vi "Save File Get File Size.vi"(8 "Error In":errorcluster, 10 "File Size":dbl=5.0 format="%#_13g", 11 "Old path":path) -> (0 "Error Out":errorcluster, 2 "File Size MB":dbl, 3 "File Size Greater Than Limit":bool)   [LabVIEW 2016, in "Save File.lvlib"]
uses:
  Save File.lvlib
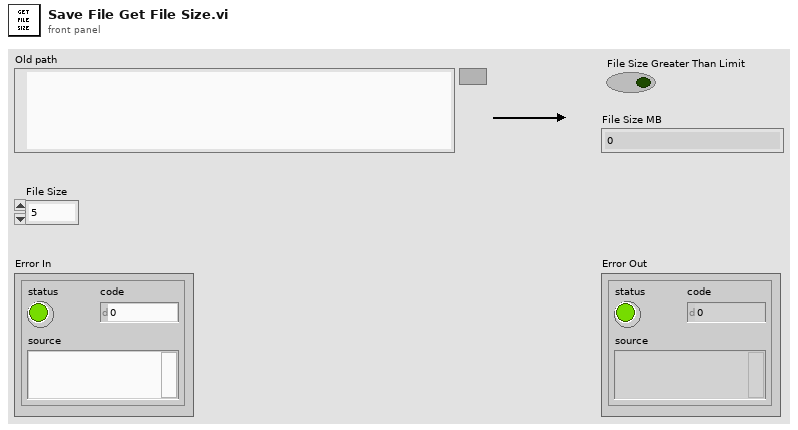
[diagram p1: front panel]
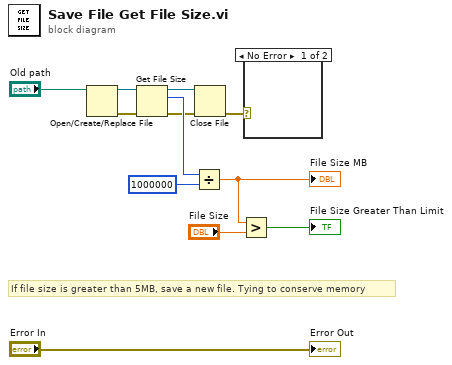
[diagram p0: block diagram]
diagram:
  # "If file size is greater than 5MB, save a new file. Tying to conserve memory"
  n1 = Open/Create/Replace File(file path (use dialog)="Old path") -> (refnum out=w3:refnum<file>, error out=w4:errorcluster)  [unwired: 5 in, 1 out]
  n2 = Get File Size(file=w3, error in=w4) -> (refnum out=w6:refnum<file>, size (in bytes)=w8:i64, 0:w5:errorcluster)
  n3 = Divide(x=w8, y=i64 1000000) -> (x/y=w11:dbl)
  "File Size MB" <- w11
  n4 = Close File(refnum=w6, error in=w5) -> (error out=w2:errorcluster)  [unwired: 1 out]
  n5 = Greater?(x=w11, y="File Size") -> (0:→"File Size Greater Than Limit":bool)
  n6 = case shown="No Error" w2 {
    frame No Error {
    }
    frame Error {
    }
  }
  "Error Out" <- "Error In"
